vi "ReadFolderConfiguration.vi"(8 "Error In":errorcluster, 11 "ABLE Config File Ref In":T2) -> (0 "Error Out":errorcluster, 2 "Folder Configuration":T1, 3 "ABLE Config File Ref Out":T2)   [LabVIEW 2012]
uses:
  <vilib>/Utility/config.llb/Config Data RefNum.ctl
  FolderConfiguration.ctl
  <vilib>/Utility/config.llb/Read Key (Path).vi
  <vilib>/Utility/config.llb/NI_LVConfig.lvlib
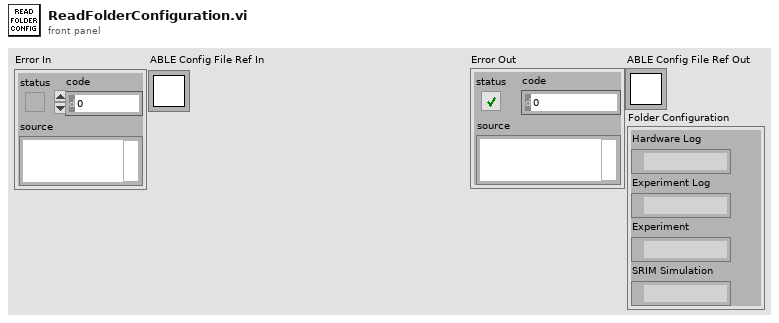
[diagram p1: front panel]
types:
  T1 = typedef "FolderConfiguration.ctl" = cluster{"Hardware Log":path, "Experiment Log":path, "Experiment":path, "SRIM Simulation":path}
  T2 = typedef "NI_LVConfig.lvlib/Config Data RefNum.ctl" = refnum<k1>
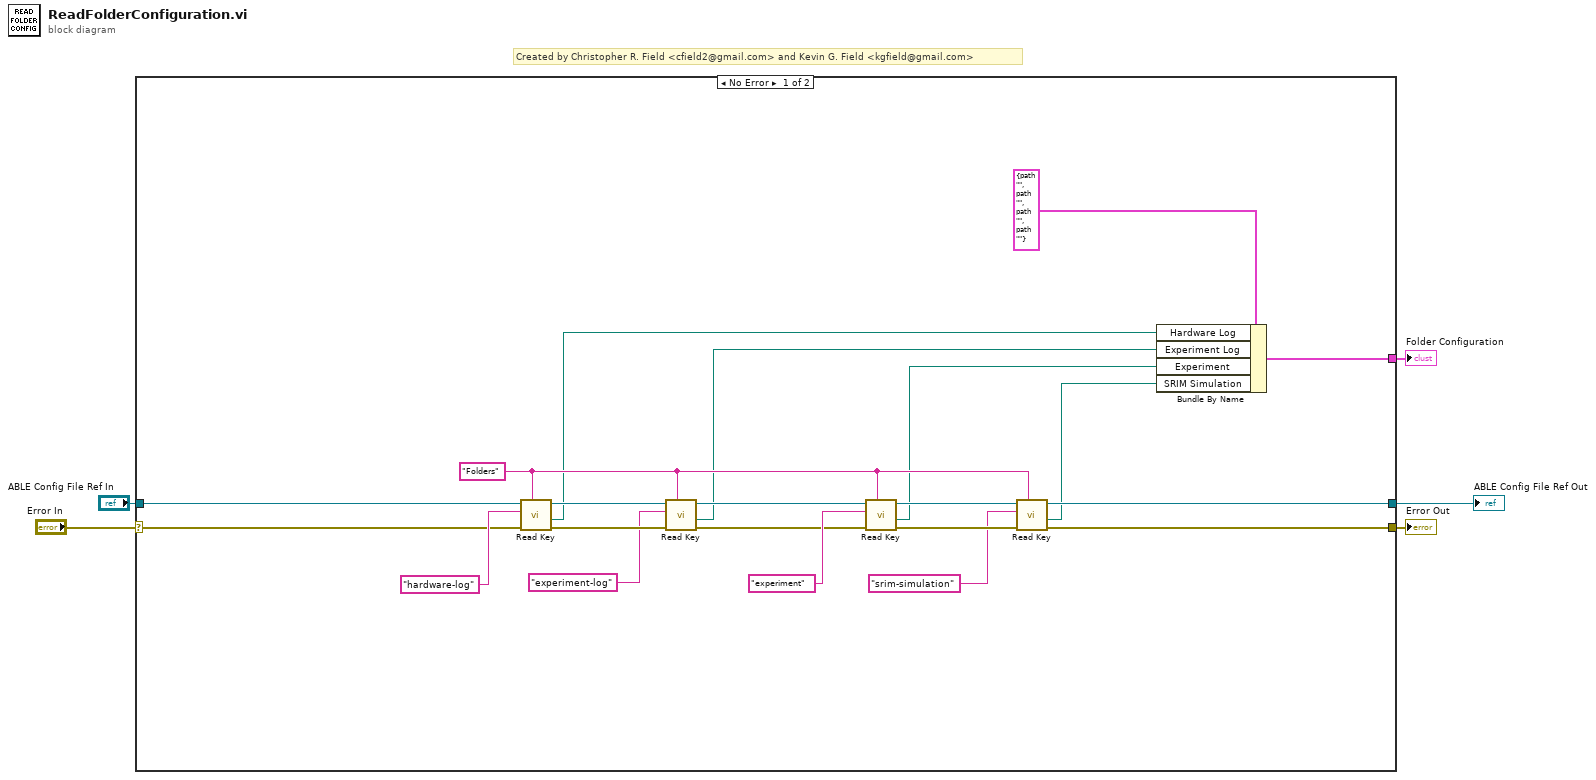
[diagram p0: block diagram]
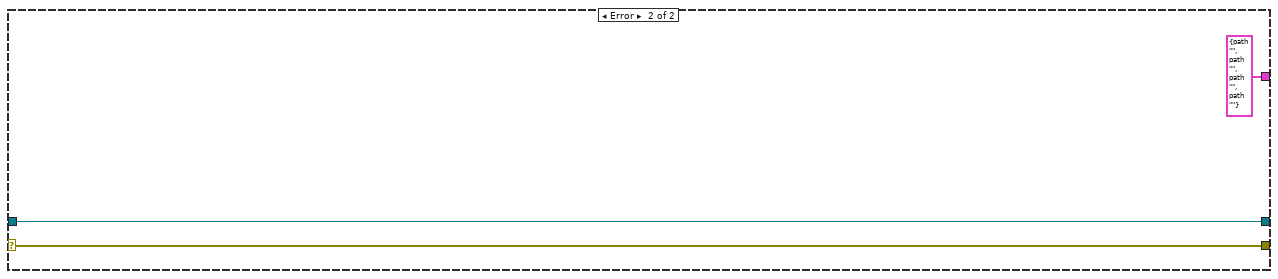
[diagram p2: hidden frame]
diagram:
  # "Created by Christopher R. Field <cfield2@gmail.com> and Kevin G. Field <kgfield@gmail.com>"
  n1 = case shown="No Error" "Error In" {
    selector: "Error In" -> [w15 w28]
    tunnel: [w14 w28] -> w4
    tunnel: [w13 w29] -> w3
    tunnel: "ABLE Config File Ref In" -> [w12 w29]
    tunnel: [w6 T1 {"Hardware Log"=path "", "Experiment Log"=path "", "Experiment"=path "", "SRIM Simulation"=path ""} ("Folder Configuration")] -> w1
    frame No Error {
      w17 = "Folders" ("section")
      n2 = call-poly <vilib>:"Read Key.vi"("section"=w17, "error in (no error)"=w15, "key"="hardware-log", "refnum"=w12) -> ("error out"=w20:errorcluster, "value"=w10:path, "refnum out"=w21:T2)  [unwired: 4 in, 1 out]
      n3 = call-poly <vilib>:"Read Key.vi"("section"=w17, "error in (no error)"=w20, "key"="experiment-log", "refnum"=w21) -> ("error out"=w18:errorcluster, "value"=w9:path, "refnum out"=w19:T2)  [unwired: 4 in, 1 out]
      n4 = call-poly <vilib>:"Read Key.vi"("section"=w17, "error in (no error)"=w18, "key"="experiment", "refnum"=w19) -> ("error out"=w23:errorcluster, "value"=w8:path, "refnum out"=w24:T2)  [unwired: 4 in, 1 out]
      n5 = call-poly <vilib>:"Read Key.vi"("section"=w17, "error in (no error)"=w23, "key"="srim-simulation", "refnum"=w24) -> ("error out"=w14:errorcluster, "value"=w7:path, "refnum out"=w13:T2)  [unwired: 4 in, 1 out]
      n6 = Bundle By Name(cluster=T1 {"Hardware Log"=path "", "Experiment Log"=path "", "Experiment"=path "", "SRIM Simulation"=path ""} ("Folder Configuration"), "Hardware Log"=w10, "Experiment Log"=w9, "Experiment"=w8, "SRIM Simulation"=w7) -> (w6:T1)
    }
    frame Error {
    }
  }
  "Error Out" <- w4
  "ABLE Config File Ref Out" <- w3
  "Folder Configuration" <- w1
